vi "Update Results.vi"(0 "MeasurementServiceV1 in":refnum<class "Measurement Service V1.lvclass">, 5 "Measurement Results":variant, 7 "MeasurementPluginService in":refnum<class "Measurement Plugin Service.lvclass">, 9 "gRPCid in":T1, 11 "error in (no error)":errorcluster) -> (4 "MeasurementServiceV1 out":refnum<class "Measurement Service V1.lvclass">, 8 "MeasurementPluginService out":refnum<class "Measurement Plugin Service.lvclass">, 15 "error out":errorcluster)   [LabVIEW 2020, in "MeasurementLink Measurement Server.lvlib" / "Measurement Service V1.lvclass"]
uses:
  Measurement Service V1.lvclass
  <vilib>/gRPC/LabVIEW gRPC Library/Shared/grpcId.ctl
  Measurement Plugin Service/Measurement Plugin Service.lvclass
  <vilib>/gRPC/LabVIEW gRPC Library/grpc-lvsupport-release.lvlib
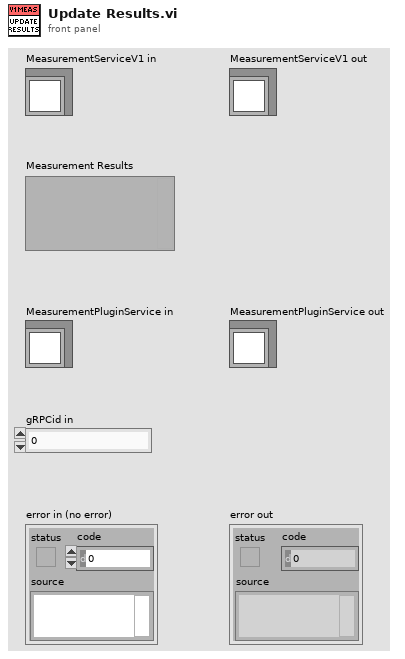
[diagram p1: front panel]
types:
  T1 = typedef "grpc-lvsupport-release.lvlib/grpcId.ctl" = u64
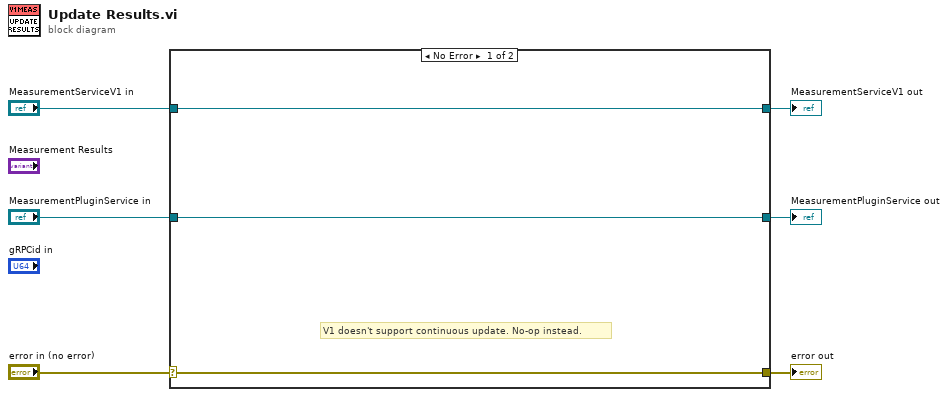
[diagram p0: block diagram]
diagram:
  n1 = case shown="No Error" "error in (no error)" {
    selector: "error in (no error)" -> [w7 w12]
    tunnel: [w7 w12] -> w5
    tunnel: [w9 w11] -> w3
    tunnel: "MeasurementServiceV1 in" -> [w9 w11]
    tunnel: "MeasurementPluginService in" -> [w8 w10]
    tunnel: [w8 w10] -> w1
    frame No Error {
      # "V1 doesn't support continuous update. No-op instead."
    }
    frame Error {
    }
  }
  "error out" <- w5
  "MeasurementServiceV1 out" <- w3
  "MeasurementPluginService out" <- w1
